vi "Exercise1.9-Case Structure.vi"() -> ()   [LabVIEW 2013]
panel:
  in  "Index":u32
  out "Output":dbl
  out "Output":dbl
  in  "Input":dbl
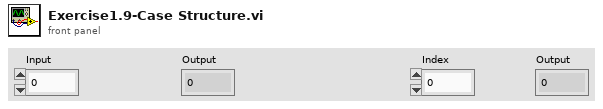
[diagram p1: front panel]
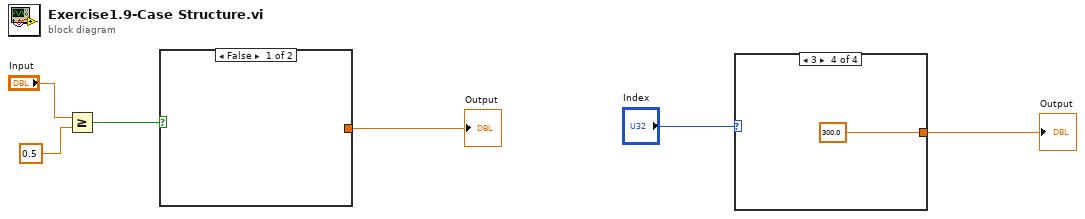
[diagram p0: block diagram]
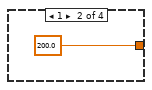
[diagram p3: hidden frame]
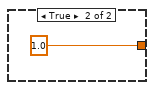
[diagram p5: hidden frame]
diagram:
  n1 = Greater Or Equal?(x="Input", y=0.5) -> (x >= y?=w6:bool)
  n2 = case shown="False" w6 {
    tunnel: [_ 1.0] -> w4
    frame False {
    }
    frame True {
    }
  }
  "Output" <- w4
  n3 = case shown="3" "Index" {
    tunnel: [_ 200.0 _ 300.0] -> w2
    frame 0, Default {
    }
    frame 1 {
    }
    frame 2 {
    }
    frame 3 {
    }
  }
  "Output" <- w2
